vi "CAN STP_Engine Stop Engine.vi"(9 "Socket No":u16, 10 "Sequence Context":T1) -> (0 "error out":errorcluster)   [LabVIEW 2023]
uses:
  <vilib>/addons/TestStand/_TSLegacy.llb/LabVIEW Test - Sequence Context.ctl
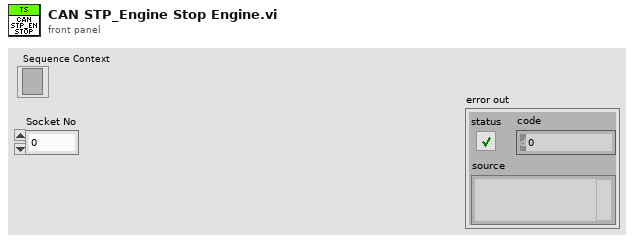
[diagram p1: front panel]
types:
  T1 = typedef "LabVIEW Test - Sequence Context.ctl" = refnum<k7>
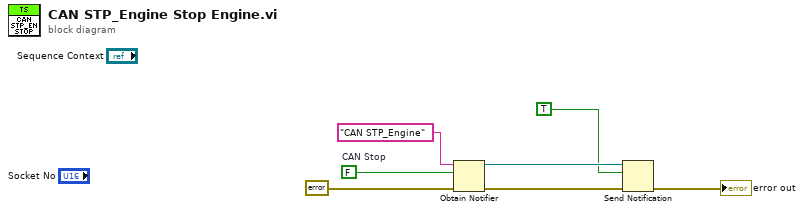
[diagram p0: block diagram]
diagram:
  w6 = FALSE  # CAN Stop
  n1 = Obtain Notifier(name (unnamed)="CAN STP_Engine", notification data type=w6, error in (no error)=errorcluster {"status"=FALSE, "code"=0, "source"=""}) -> (notifier out=w2:refnum<notifier>, error out=w4:errorcluster)  [unwired: 1 in, 1 out]
  n2 = Send Notification(notification=TRUE, notifier=w2, error in (no error)=w4) -> (error out=→"error out":errorcluster)  [unwired: 1 out]
